vi "Create.vi"(8 "error in (no error)":errorcluster, 11 "reference in":refnum<class "BasePlugin.lvclass">) -> (0 "error out":errorcluster, 3 "reference out":refnum<class "BasePlugin.lvclass">)   [LabVIEW 2014, in "BaseClasses.lvlib" / "BasePlugin.lvclass"]
uses:
  BasePlugin.lvclass
  Object_class/BaseObject.lvclass
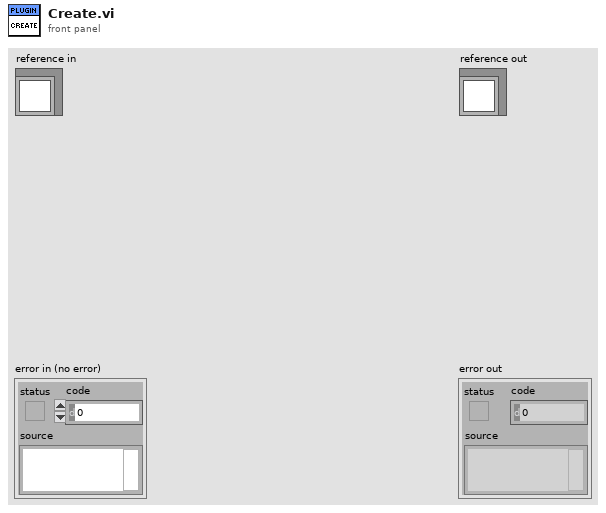
[diagram p1: front panel]
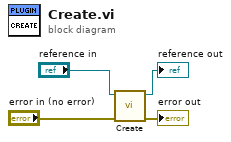
[diagram p0: block diagram]
diagram:
  n1 = call-parent "Create.vi"("error in (no error)"="error in (no error)", "reference in"="reference in") -> ("error out"=→"error out":errorcluster, "reference out"=→"reference out":refnum<class "BasePlugin.lvclass">)  [unwired: 8 in]
